vi "EN50160 Statistical Evaluation (1 week).vi"(0 "2hr values":T2(array[cluster]), 1 "evaluated data":enum16{"all data", "data without flag"}(ring), 2 "nominal frequency":enum16{"50 Hz", "60 Hz"}(ring), 5 "10min values":T5(array[cluster]), 7 "10sec values":T4(array[cluster]), 9 "3sec values":T3(array[cluster]), 11 "error in (no error)":errorcluster, 12 "nominal voltage [V]":dbl=230.0, 13 "signaling frequency [Hz]":dbl=216.66) -> (4 "EN50160 results":T1, 10 "all passed?":bool, 15 "error out":errorcluster)   [LabVIEW 2014, in "NI_EP_Power Quality.lvlib"]
doc: "Performs a statistical evaluation of one week aggregated data to evaluate whether the data satisfies the normal operation conditions defined by EN50160."
uses:
  <vilib>/addons/Electrical Power/PQ/NI_EP_Power Quality.lvlib
  <vilib>/addons/Electrical Power/PQ/Utility/subVIs/ep_EN50160 Basic Statistical Evaluation (1D).vi
  <vilib>/addons/Electrical Power/PQ/Utility/subVIs/ep_EN50160 Basic Statistical Evaluation (2D).vi
  <vilib>/addons/Electrical Power/PQ/Utility/subVIs/ep_EN50160 Basic Statistical Evaluation (3D).vi
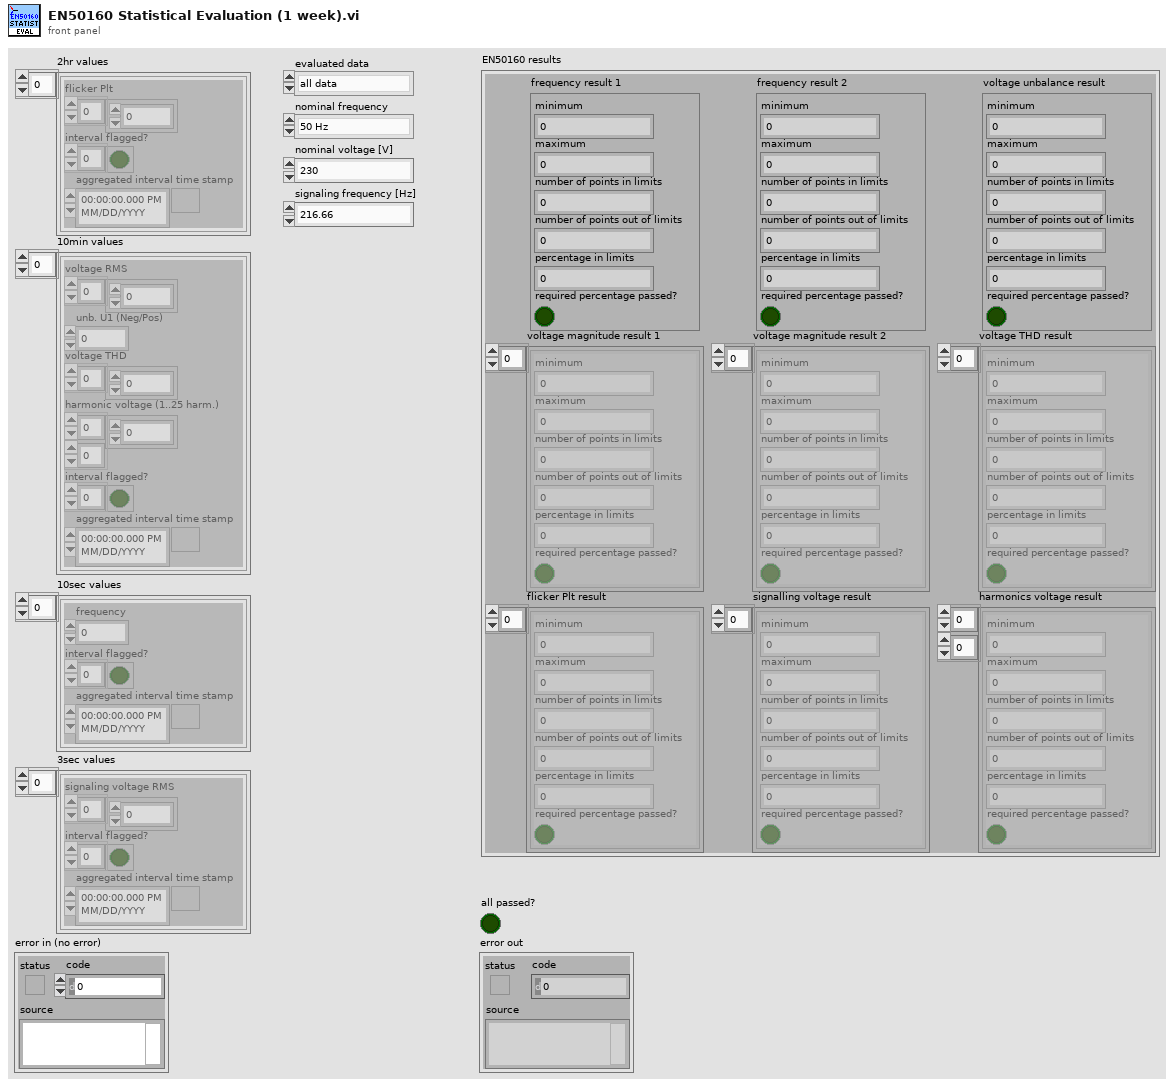
[diagram p1: front panel]
types:
  T1 = cluster{"frequency result 1":cluster{"minimum":dbl, "maximum":dbl, "number of points in limits":u32, "number of points out of limits":u32, "percentage in limits":dbl, "required percentage passed?":bool}, "frequency result 2":cluster{"minimum":dbl, "maximum":dbl, "number of points in limits":u32, "number of points out of limits":u32, "percentage in limits":dbl, "required percentage passed?":bool}, "voltage magnitude result 1":cluster{"minimum":dbl, "maximum":dbl, "number of points in limits":u32, "number of points out of limits":u32, "percentage in limits":dbl, "required percentage passed?":bool}[], "voltage magnitude result 2":cluster{"minimum":dbl, "maximum":dbl, "number of points in limits":u32, "number of points out of limits":u32, "percentage in limits":dbl, "required percentage passed?":bool}[], "flicker Plt result":cluster{"minimum":dbl, "maximum":dbl, "number of points in limits":u32, "number of points out of limits":u32, "percentage in limits":dbl, "required percentage passed?":bool}[], "signalling voltage result":cluster{"minimum":dbl, "maximum":dbl, "number of points in limits":u32, "number of points out of limits":u32, "percentage in limits":dbl, "required percentage passed?":bool}[], "voltage unbalance result":cluster{"minimum":dbl, "maximum":dbl, "number of points in limits":u32, "number of points out of limits":u32, "percentage in limits":dbl, "required percentage passed?":bool}, "voltage THD result":cluster{"minimum":dbl, "maximum":dbl, "number of points in limits":u32, "number of points out of limits":u32, "percentage in limits":dbl, "required percentage passed?":bool}[], "harmonics voltage result":cluster{"minimum":dbl, "maximum":dbl, "number of points in limits":u32, "number of points out of limits":u32, "percentage in limits":dbl, "required percentage passed?":bool}[][]}
  T2 = cluster{"flicker Plt":dbl[], "interval flagged?":bool[], "aggregated interval time stamp":timestamp}[]
  T3 = cluster{"signaling voltage RMS":dbl[], "interval flagged?":bool[], "aggregated interval time stamp":timestamp}[]
  T4 = cluster{"frequency":dbl, "interval flagged?":bool[], "aggregated interval time stamp":timestamp}[]
  T5 = cluster{"voltage RMS":dbl[], "unb. U1 (Neg/Pos)":dbl, "voltage THD":dbl[], "harmonic voltage (1..25 harm.)":dbl[][], "interval flagged?":bool[], "aggregated interval time stamp":timestamp}[]
  T6 = cluster{"frequency limits 1":cluster{"upper limit":dbl, "lower limit":dbl, "required percentage":dbl}, "frequency limits 2":cluster{"upper limit":dbl, "lower limit":dbl, "required percentage":dbl}, "voltage magnitude limits 1":cluster{"upper limit":dbl, "lower limit":dbl, "required percentage":dbl}, "voltage magnitude limits 2":cluster{"upper limit":dbl, "lower limit":dbl, "required percentage":dbl}, "flicker Plt limits":cluster{"upper limit":dbl, "lower limit":dbl, "required percentage":dbl}, "signalling voltage limits":cluster{"upper limit":dbl, "lower limit":dbl, "required percentage":dbl}, "voltage unbalance limits":cluster{"upper limit":dbl, "lower limit":dbl, "required percentage":dbl}, "voltage THD limits":cluster{"upper limit":dbl, "lower limit":dbl, "required percentage":dbl}, "harmonics voltage limits (1..25 harm.)":cluster{"upper limit":dbl, "lower limit":dbl, "required percentage":dbl}[]}
  T7 = cluster{"upper limit":dbl, "lower limit":dbl, "required percentage":dbl}
  T8 = cluster{"upper limit":dbl, "lower limit":dbl, "required percentage":dbl}[]
  T9 = cluster{"minimum":dbl, "maximum":dbl, "number of points in limits":u32, "number of points out of limits":u32, "percentage in limits":dbl, "required percentage passed?":bool}
  T10 = cluster{"minimum":dbl, "maximum":dbl, "number of points in limits":u32, "number of points out of limits":u32, "percentage in limits":dbl, "required percentage passed?":bool}[]
  T11 = cluster{"minimum":dbl, "maximum":dbl, "number of points in limits":u32, "number of points out of limits":u32, "percentage in limits":dbl, "required percentage passed?":bool}[][]
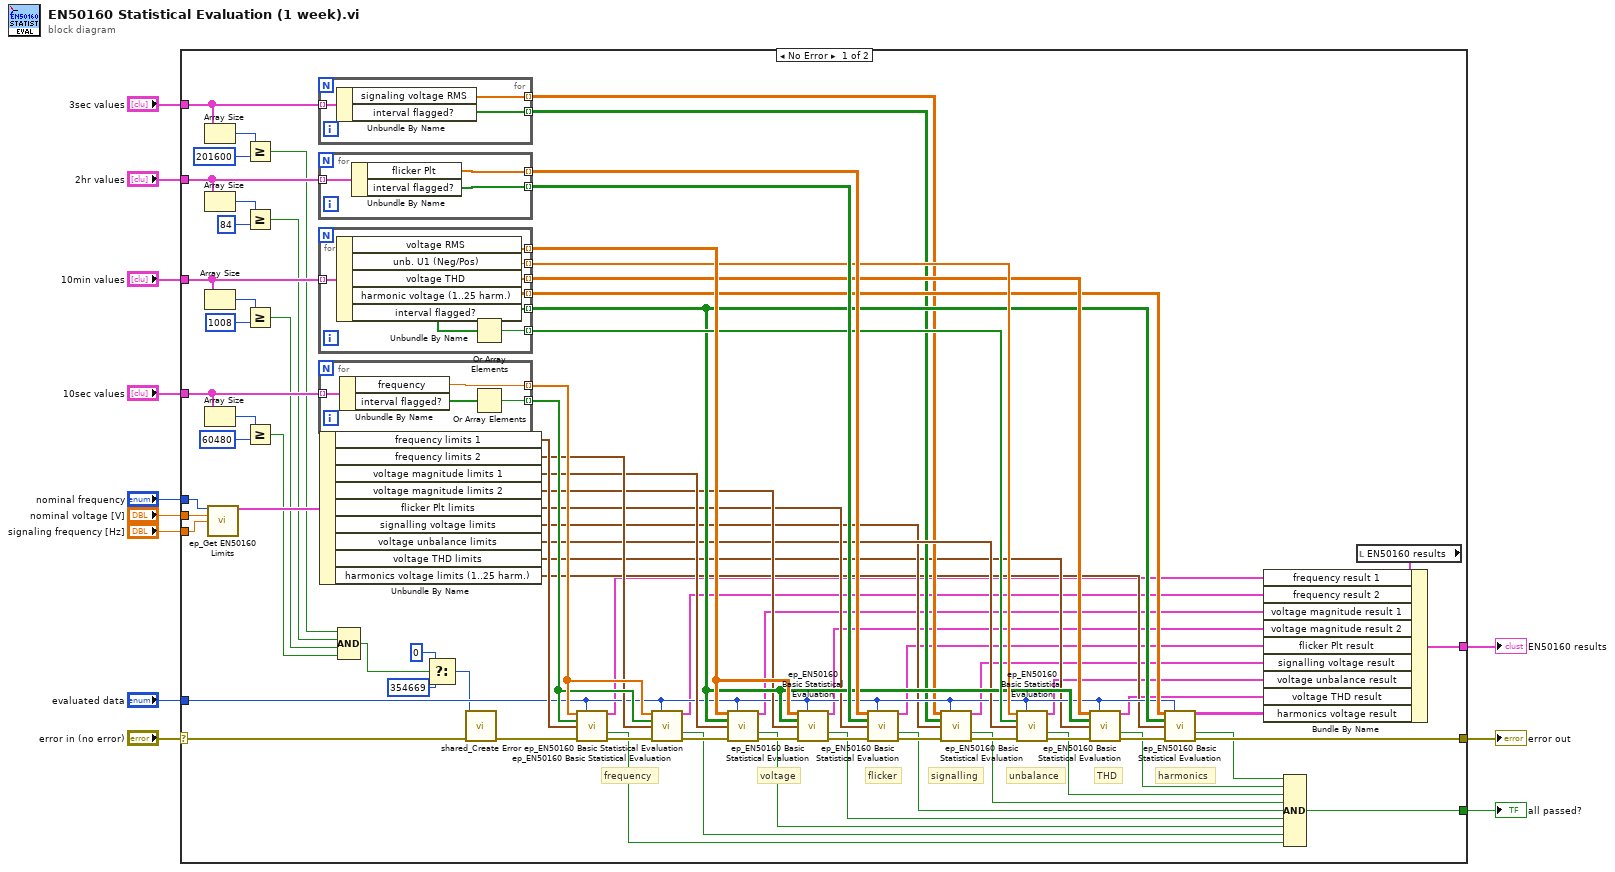
[diagram p0: block diagram]
diagram:
  n1 = case shown="No Error" "error in (no error)" {
    selector: "error in (no error)" -> [w14 w108]
    tunnel: [w58 w108] -> w11
    tunnel: "evaluated data" -> [w62 _]
    tunnel: "10min values" -> [w24 _]
    tunnel: "10sec values" -> [w25 _]
    tunnel: "nominal frequency" -> [w72 _]
    tunnel: "3sec values" -> [w34 _]
    tunnel: "nominal voltage [V]" -> [w73 _]
    tunnel: "2hr values" -> [w23 _]
    tunnel: "signaling frequency [Hz]" -> [w74 _]
    tunnel: [w52 _] -> w2
    tunnel: [w35 _] -> w1
    frame No Error {
      # "signalling"
      # "harmonics"
      # "THD"
      # "unbalance"
      # "flicker"
      # "voltage"
      # "frequency"
      n2 = Array Size(array=w34) -> (size(s)=w33:i32)
      n3 = Array Size(array=w23) -> (size(s)=w30:i32)
      n4 = Array Size(array=w24) -> (size(s)=w29:i32)
      n5 = Array Size(array=w25) -> (size(s)=w26:i32)
      n6 = call <vilib>:"ep_Get EN50160 Limits.vi"("nominal frequency"=w72, "nominal voltage [V]"=w73, "signaling frequency [Hz]"=w74) -> ("EN50160 limits"=w71:T6)  [unwired: 12 in]
      n7 = Greater Or Equal?(x=w33, y=201600) -> (x >= y?=w22:bool)
      n8 = Greater Or Equal?(x=w30, y=84) -> (x >= y?=w21:bool)
      n9 = Greater Or Equal?(x=w29, y=1008) -> (x >= y?=w20:bool)
      n10 = Greater Or Equal?(x=w26, y=60480) -> (x >= y?=w19:bool)
      n11 = for {
        tunnel: w34 -> [w96] mode=indexing
        tunnel: [w95] -> w61 mode=indexing
        tunnel: [w94] -> w60 mode=indexing
        n12 = Unbundle By Name(w96) -> ("signaling voltage RMS"=w95:dbl[], "interval flagged?"=w94:bool[])
      }
      n13 = for {
        tunnel: w23 -> [w93] mode=indexing
        tunnel: [w92] -> w83 mode=indexing
        tunnel: [w91] -> w82 mode=indexing
        n14 = Unbundle By Name(w93) -> ("flicker Plt"=w92:dbl[], "interval flagged?"=w91:bool[])
      }
      n15 = for {
        tunnel: w24 -> [w107] mode=indexing
        tunnel: [w106] -> w84 mode=indexing
        tunnel: [w105] -> w81 mode=indexing
        tunnel: [w104] -> w78 mode=indexing
        tunnel: [w103] -> w76 mode=indexing
        tunnel: [w102] -> w75 mode=indexing
        tunnel: [w101] -> w80 mode=indexing
        n16 = Unbundle By Name(w107) -> ("voltage RMS"=w106:dbl[], "unb. U1 (Neg/Pos)"=w105:dbl, "voltage THD"=w104:dbl[], "harmonic voltage (1..25 harm.)"=w103:dbl[][], "interval flagged?"=w102:bool[])
        n17 = Or Array Elements(Boolean array=w102) -> (logical OR=w101:bool)
      }
      n18 = for {
        tunnel: w25 -> [w100] mode=indexing
        tunnel: [w99] -> w89 mode=indexing
        tunnel: [w97] -> w88 mode=indexing
        n19 = Unbundle By Name(w100) -> ("frequency"=w99:dbl, "interval flagged?"=w98:bool[])
        n20 = Or Array Elements(Boolean array=w98) -> (logical OR=w97:bool)
      }
      n21 = Unbundle By Name(w71) -> ("frequency limits 1"=w70:T7, "frequency limits 2"=w69:T7, "voltage magnitude limits 1"=w68:T7, "voltage magnitude limits 2"=w67:T7, "flicker Plt limits"=w66:T7, "signalling voltage limits"=w59:T7, "voltage unbalance limits"=w65:T7, "voltage THD limits"=w57:T7, "harmonics voltage limits (1..25 harm.)"=w56:T8)
      n22 = Compound Arithmetic op=AND(w22, w21, w20, w19) -> (w18:bool)
      n23 = Select(t=0 ("error code (0)"), s=w18, f=354669) -> (s? t:f=w15:i32)
      n24 = call <vilib>:"shared_Create Error.vi"("error in (no error)"=w14, "error code (0)"=w15) -> ("error out"=w13:errorcluster)  [unwired: 9 in]
      n25 = call-poly <vilib>:"ep_EN50160 Basic Statistical Evaluation.vi"("data"=w89, "evaluated data"=w62, "data flags"=w88, "EN50160 limits"=w70, "error in (no error)"=w13) -> ("EN50160 result"=w45:T9, "passed?"=w36:bool, "error out"=w90:errorcluster)  [unwired: 8 in]
      n26 = call-poly <vilib>:"ep_EN50160 Basic Statistical Evaluation.vi"("data"=w89, "evaluated data"=w62, "data flags"=w88, "EN50160 limits"=w69, "error in (no error)"=w90) -> ("EN50160 result"=w46:T9, "passed?"=w37:bool, "error out"=w86:errorcluster)  [unwired: 8 in]
      n27 = call-poly <vilib>:"ep_EN50160 Basic Statistical Evaluation.vi"("data"=w84, "evaluated data"=w62, "data flags"=w75, "EN50160 limits"=w68, "error in (no error)"=w86) -> ("EN50160 results"=w47:T10, "passed?"=w38:bool, "error out"=w87:errorcluster)  [unwired: 8 in]
      n28 = call-poly <vilib>:"ep_EN50160 Basic Statistical Evaluation.vi"("data"=w84, "evaluated data"=w62, "data flags"=w75, "EN50160 limits"=w67, "error in (no error)"=w87) -> ("EN50160 results"=w48:T10, "passed?"=w39:bool, "error out"=w85:errorcluster)  [unwired: 8 in]
      n29 = call-poly <vilib>:"ep_EN50160 Basic Statistical Evaluation.vi"("data"=w83, "evaluated data"=w62, "data flags"=w82, "EN50160 limits"=w66, "error in (no error)"=w85) -> ("EN50160 results"=w49:T10, "passed?"=w40:bool, "error out"=w64:errorcluster)  [unwired: 8 in]
      n30 = call-poly <vilib>:"ep_EN50160 Basic Statistical Evaluation.vi"("data"=w61, "evaluated data"=w62, "data flags"=w60, "EN50160 limits"=w59, "error in (no error)"=w64) -> ("EN50160 results"=w50:T10, "passed?"=w41:bool, "error out"=w63:errorcluster)  [unwired: 8 in]
      n31 = call-poly <vilib>:"ep_EN50160 Basic Statistical Evaluation.vi"("data"=w81, "evaluated data"=w62, "data flags"=w80, "EN50160 limits"=w65, "error in (no error)"=w63) -> ("EN50160 result"=w51:T9, "passed?"=w42:bool, "error out"=w79:errorcluster)  [unwired: 8 in]
      n32 = call-poly <vilib>:"ep_EN50160 Basic Statistical Evaluation.vi"("data"=w78, "evaluated data"=w62, "data flags"=w75, "EN50160 limits"=w57, "error in (no error)"=w79) -> ("EN50160 results"=w53:T10, "passed?"=w43:bool, "error out"=w77:errorcluster)  [unwired: 8 in]
      n33 = call-poly <vilib>:"ep_EN50160 Basic Statistical Evaluation.vi"("data"=w76, "evaluated data"=w62, "data flags"=w75, "EN50160 limits"=w56, "error in (no error)"=w77) -> ("EN50160 results"=w55:T11, "passed?"=w44:bool, "error out"=w58:errorcluster)  [unwired: 8 in]
      n34 = Compound Arithmetic op=AND(w44, w43, w42, w41, w40, w39, w38, w37, w36) -> (w35:bool)
      n35 = local read "EN50160 results"() -> (w54:T1)
      n36 = Bundle By Name(cluster=w54, "frequency result 1"=w45, "frequency result 2"=w46, "voltage magnitude result 1"=w47, "voltage magnitude result 2"=w48, "flicker Plt result"=w49, "signalling voltage result"=w50, "voltage unbalance result"=w51, "voltage THD result"=w53, "harmonics voltage result"=w55) -> (w52:T1)
    }
    frame Error {
    }
  }
  "error out" <- w11
  "EN50160 results" <- w2
  "all passed?" <- w1
